vi "Set start buttons enabling state.vi"(8 "error in (no error)":errorcluster, 11 "DAQOrcaFlash in":refnum<class "DAQOrcaFlash.lvclass">) -> (0 "error out":errorcluster, 3 "DAQOrcaFlash out":refnum<class "DAQOrcaFlash.lvclass">)   [LabVIEW 2012, in "DAQOrcaFlash.lvclass"]
uses:
  DAQOrcaFlash.lvclass
  DAQOrcaFlash.lvclass/DAQOrcaFlash.ctl
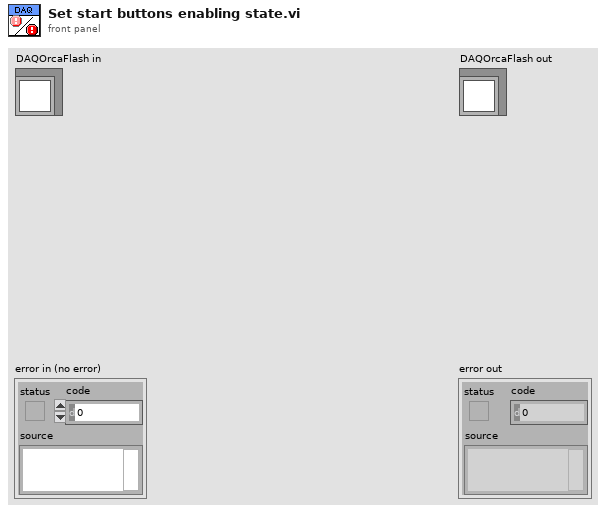
[diagram p1: front panel]
types:
  T1 = enum8{"Enabled", "Disabled", "Disabled and Grayed Out"}
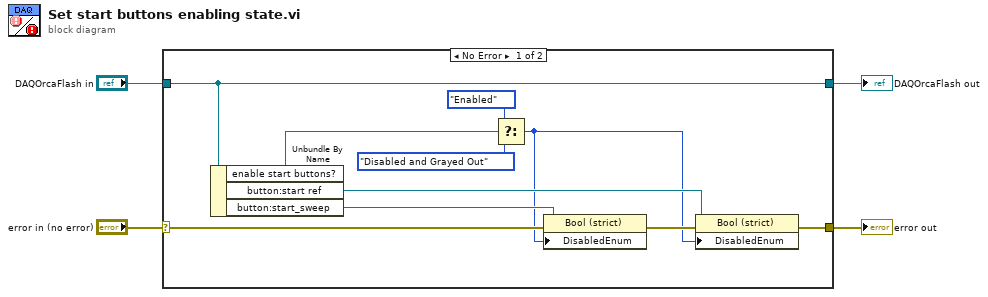
[diagram p0: block diagram]
diagram:
  n1 = case shown="No Error" "error in (no error)" {
    selector: "error in (no error)" -> [w7 w16]
    tunnel: [w6 w16] -> w3
    tunnel: [w14 w15] -> w1
    tunnel: "DAQOrcaFlash in" -> [w14 w15]
    frame No Error {
      n2 = Unbundle By Name(w14) -> ("enable start buttons?"=w12:bool, "button:start ref"=w13:refnum<vi>, "button:start_sweep"=w9:refnum<vi>)
      n3 = Select(t=T1."Enabled" ("Disabled"), s=w12, f=T1."Disabled and Grayed Out" ("Disabled")) -> (s? t:f=w5:T1)
      n4 = property class="Bool (strict)"(reference=w9, error in=w7, "DisabledEnum"=w5) -> (error out=w8:errorcluster)  [unwired: 1 out]
      n5 = property class="Bool (strict)"(reference=w13, error in=w8, "DisabledEnum"=w5) -> (error out=w6:errorcluster)  [unwired: 1 out]
    }
    frame Error {
    }
  }
  "error out" <- w3
  "DAQOrcaFlash out" <- w1
